vi "light.vi"() -> ()   [LabVIEW 2015]
uses:
  <vilib>/NXT/Block Support/NXT_InputPort.ctl
  <vilib>/NXT/Block Support/NXT_OutputPort.ctl
  <vilib>/NXT/Dual Mode Library/Sensors/Light_On.vi
  <vilib>/NXT/NXTIO Xnodes/NXTIONodeSubVIs/NXTMoveMotors.vi
  <vilib>/NXT/NXTIO Xnodes/AddressXNode/NXTIOAddress.xnode
  <vilib>/NXT/Subs/LVHSConnector.ctl
  <vilib>/NXT/NXTIO Xnodes/NXTIOXNode/NXTIO.xnode
  <vilib>/NXT/LegoClasses/BrickReference/BrickReference.lvclass
panel:
  in  "stop":bool
  in  "Port (Port 3)":T1=2 items=["Port 1", "Port 2", "Port 3", "Port 4"]
  in  "Power/Speed 1":i8=75
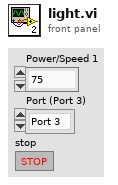
[diagram p1: front panel]
types:
  T1 = typedef "NXT_InputPort.ctl" = u32
  T2 = typedef "NXT_OutputPort.ctl" = u8
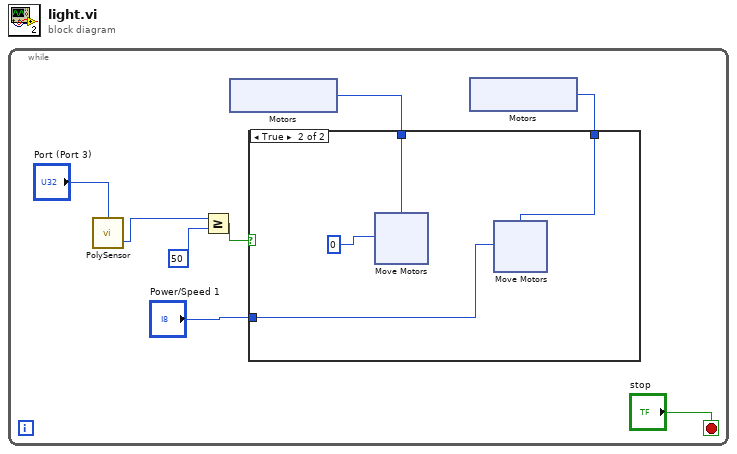
[diagram p0: block diagram]
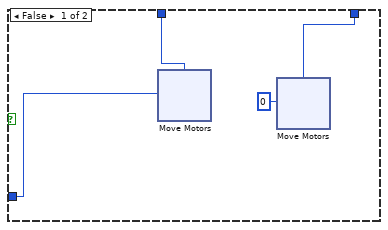
[diagram p2: hidden frame]
diagram:
  n1 = while {
    stop <- "stop" stop-if-true
    n2 = call-poly <vilib>:"PolySensor.vi"("Port (Port 3)"="Port (Port 3)") -> ("Scaled Value"=w6:i16)  [unwired: 2 in, 1 out]
    n3 = Greater Or Equal?(x=w6, y=50) -> (x >= y?=w4:bool)
    n4 = xnode "Motors"() -> ("Motor"=w3:T2)
    n5 = xnode "Motors"() -> ("Motor"=w2:T2)
    n6 = case shown="True" w4 {
      tunnel: "Power/Speed 1" -> [w12 w31]
      tunnel: w3 -> [w14 w30]
      tunnel: w2 -> [w13 w29]
      frame False {
        n7 = xnode "Move Motors"("Power/Speed 1"=w12, "Motors"=w14) -> ()  [unwired: 1 in, 1 out]
        n8 = xnode "Move Motors"("Power/Speed 1"=i8 0, "Motors"=w13) -> ()  [unwired: 1 in, 1 out]
      }
      frame True {
        n9 = xnode "Move Motors"("Power/Speed 1"=0, "Motors"=w30) -> ()  [unwired: 1 in, 1 out]
        n10 = xnode "Move Motors"("Power/Speed 1"=w31, "Motors"=w29) -> ()  [unwired: 1 in, 1 out]
      }
    }
  }
